vi "Self-Test.vi"(8 "error in (no error)":errorcluster {"code" format="%.0x"}, 11 "instrument handle":refnum<k15>) -> (0 "error out":errorcluster {"code" format="%.0x"}, 1 "self-test message":string, 2 "self test result":i16 format="%.0g", 3 "instrument handle out":refnum<k15>)   [LabVIEW 2021, in "Keysight XSAnVMA.lvlib"]
doc: "Performs an instrument self test, waits for the instrument to complete the test, and queries the instrument for the results. If the instrument passes the test, TestResult is zero and TestMessage is 'Self test passed'."
uses:
  <instrlib>/Keysight XSAnVMA/Keysight XSAnVMA.lvlib
  KtXSAnVMA_64.dll
panel:
  in  "Buffer size":i32=256
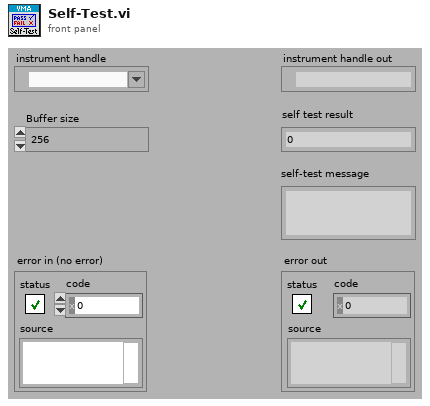
[diagram p1: front panel]
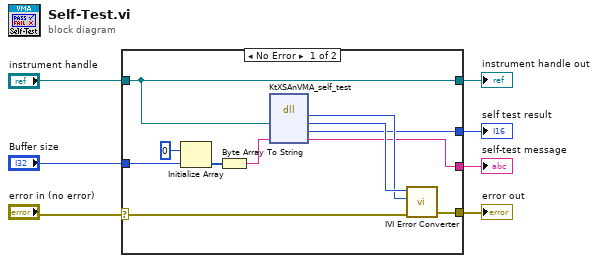
[diagram p0: block diagram]
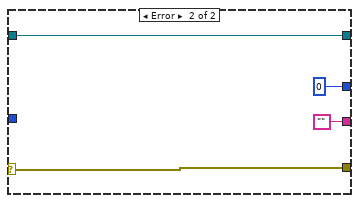
[diagram p2: hidden frame]
diagram:
  n1 = case shown="No Error" "error in (no error)" {
    selector: "error in (no error)" -> [w11 w19]
    tunnel: [w14 w19] -> w7
    tunnel: "instrument handle" -> [w12 w22]
    tunnel: [w12 w22] -> w5
    tunnel: [w10 i16 0 ("self test result")] -> w3
    tunnel: [w9 ""] -> w2
    tunnel: "Buffer size" -> [w8 _]
    frame No Error {
      n2 = Initialize Array(u8 0, w8) -> (w17:u8[])
      n3 = Byte Array To String(unsigned byte array=w17) -> (string=w16:string)
      n4 = dll-call lib="KtXSAnVMA**.dll" fn="KtXSAnVMA_self_test" ("LabVIEW:IviDmm_self_test")("instrument handle"=w12, "self-test message"=w16) -> ("Status"=w13:i32, "instrument handle"=w15:u32, "self test result"=w10:i16, "self-test message"=w9:string)  [unwired: 3 in, 3 out]
      n5 = call <instrlib>:"IVI Error Converter.vi"("error in (no error)"=w11, "IVI error code (0)"=w13, "instrument handle"=w15) -> ("error out"=w14:errorcluster)  [unwired: 7 in, 1 out]
    }
    frame Error {
    }
  }
  "error out" <- w7
  "instrument handle out" <- w5
  "self test result" <- w3
  "self-test message" <- w2
